vi "FxSine.vi"(4 "相位":dbl, 6 "偏移":dbl, 7 "采样频率":dbl=200.0, 8 "幅值":dbl, 9 "频率":dbl, 10 "终点时间":dbl, 11 "起点时间":dbl) -> (0 "Y":dbl[](array[numeric]), 3 "X":dbl[](array[numeric]))   [LabVIEW 2020, in "Curve Editor.lvlib"]
uses:
  Curve Editor.lvlib
panel:
  out "XY图":cluster{dbl[], dbl[]}(graph)
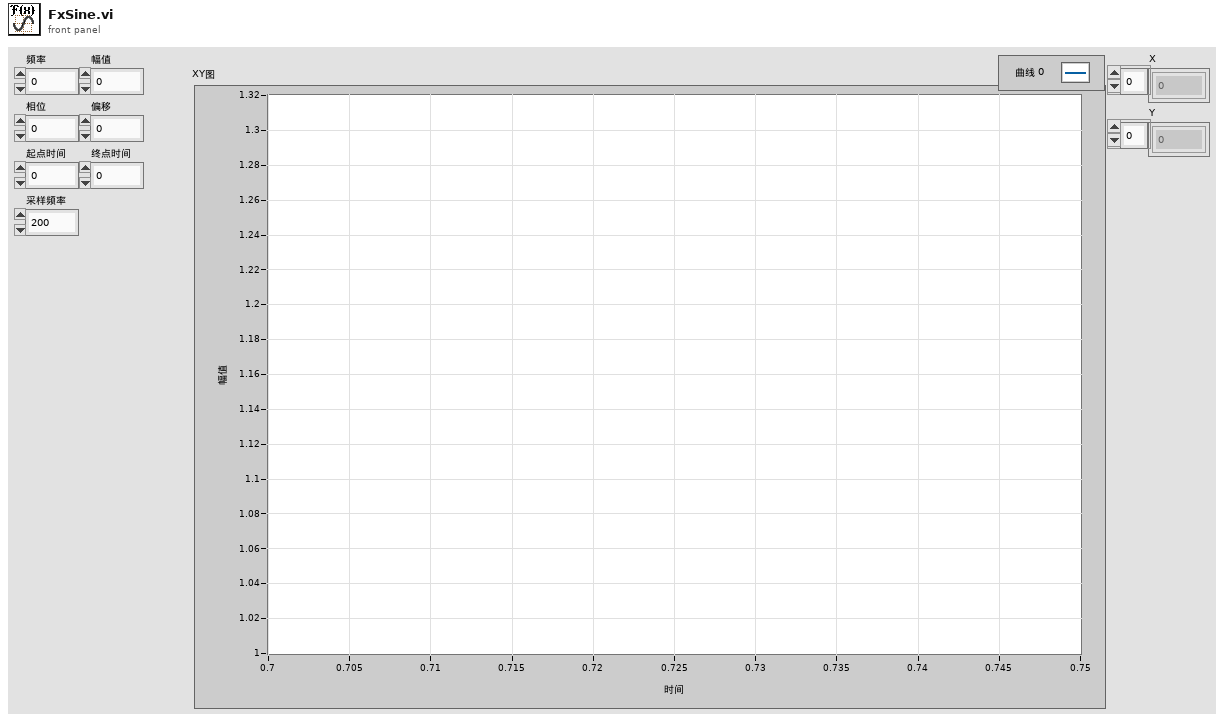
[diagram p1: front panel]
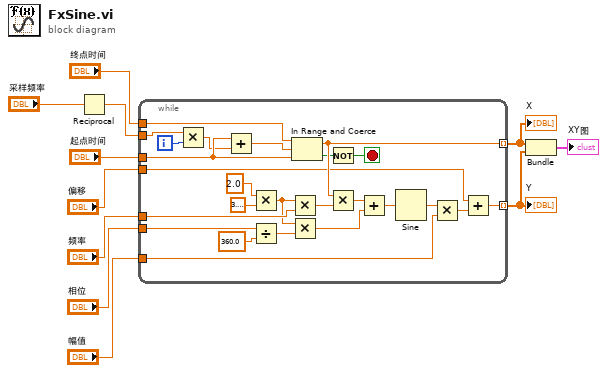
[diagram p0: block diagram]
diagram:
  n1 = Reciprocal(x="采样频率") -> (1/x=w5:dbl)
  n2 = while {
    tunnel: "频率" -> [w34]
    tunnel: [w24] -> w9 mode=indexing
    tunnel: [w17] -> w10 mode=indexing
    tunnel: "起点时间" -> [w22]
    tunnel: "终点时间" -> [w23]
    tunnel: w5 -> [w19]
    tunnel: "相位" -> [w14]
    tunnel: "幅值" -> [w13]
    tunnel: "偏移" -> [w12]
    i -> [w21]
    stop <- w15 stop-if-true
    n3 = Multiply(x=w19, y=w21) -> (x*y=w20:dbl)
    n4 = Add(x=w22, y=w20) -> (x+y=w18:dbl)
    n5 = Multiply(x=2.0, y=3.141592653589793) -> (x*y=w31:dbl)
    n6 = Divide(x=w14, y=360.0) -> (x/y=w32:dbl)
    n7 = Multiply(x=w31, y=w34) -> (x*y=w27:dbl)
    n8 = Multiply(x=w31, y=w32) -> (x*y=w30:dbl)
    n9 = In Range and Coerce(upper limit=w23, x=w18, lower limit=w22) -> (coerced(x)=w17:dbl, In Range?=w16:bool)
    n10 = Not(x=w16) -> (.not. x?=w15:bool)
    n11 = Multiply(x=w17, y=w27) -> (x*y=w26:dbl)
    n12 = Add(x=w26, y=w30) -> (x+y=w29:dbl)
    n13 = Sine(x=w29) -> (sin(x)=w28:dbl)
    n14 = Multiply(x=w28, y=w13) -> (x*y=w25:dbl)
    n15 = Add(x=w12, y=w25) -> (x+y=w24:dbl)
  }
  "X" <- w10
  "Y" <- w9
  n16 = Bundle(w10, w9) -> (→"XY图":cluster{dbl[], dbl[]})  [unwired: 1 in]
